vi "readPDO.vi"(8 "error in (no error)":errorcluster, 9 "TPDO object in":refnum<k20>, 11 "Orion_BMS in":refnum<class "Orion_BMS.lvclass">) -> (0 "error out":errorcluster, 1 "TPDO object out":refnum<k20>, 2 "TPDO data":u8[](array[numeric]), 3 "Orion_BMS out":refnum<class "Orion_BMS.lvclass">, 5 "new data?":bool)   [LabVIEW 2018, in "Orion_BMS.lvclass"]
uses:
  Orion_BMS.lvclass
  Orion_BMS.lvclass/Orion_BMS.ctl
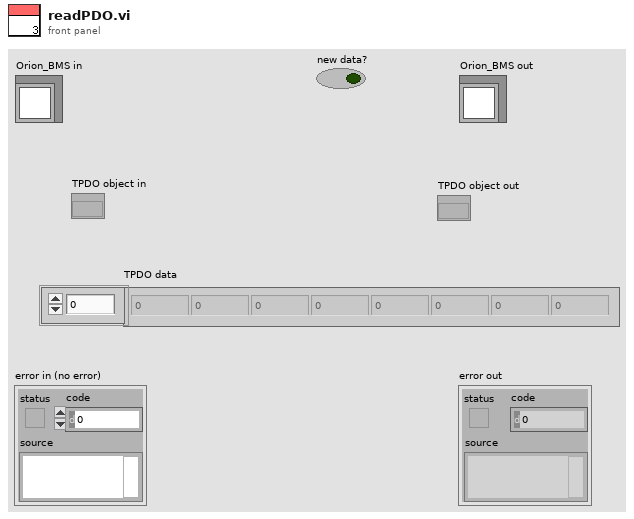
[diagram p1: front panel]
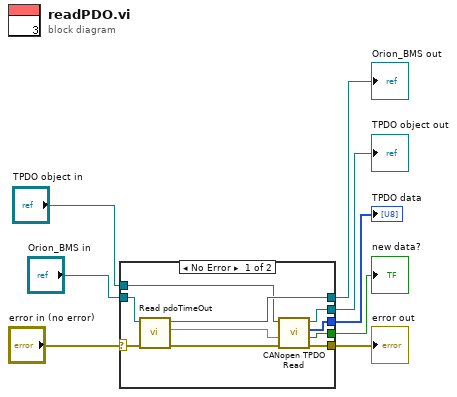
[diagram p0: block diagram]
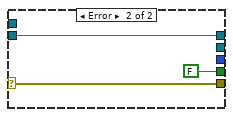
[diagram p2: hidden frame]
diagram:
  n1 = case shown="No Error" "error in (no error)" {
    selector: "error in (no error)" -> [w13 w21]
    tunnel: [w10 w21] -> w7
    tunnel: [w16 w20] -> w5
    tunnel: "Orion_BMS in" -> [w12 w20]
    tunnel: [w15 _] -> w4
    tunnel: [w14 FALSE ("new data?")] -> w3
    tunnel: "TPDO object in" -> [w11 _]
    tunnel: [w9 _] -> w1
    frame No Error {
      n2 = call "Read pdoTimeOut.vi"("error in (no error)"=w13, "OrionBMS in"=w12) -> ("error out"=w17:errorcluster, "pdoTimeOut"=w18:dbl, "OrionBMS out"=w16:refnum<class "Orion_BMS.lvclass">)  [unwired: 7 in]
      n3 = call <vilib>:"CANopen TPDO Read.vi"("error in (no error)"=w17, "timeout (0s)"=w18, "TPDO object in"=w11) -> ("error out"=w10:errorcluster, "new data?"=w14:bool, "data"=w15:u8[], "TPDO object out"=w9:refnum<k20>)  [unwired: 4 in, 1 out]
    }
    frame Error {
    }
  }
  "error out" <- w7
  "Orion_BMS out" <- w5
  "TPDO data" <- w4
  "new data?" <- w3
  "TPDO object out" <- w1
